vi "test2.vi"() -> ()   [LabVIEW 2025]
panel:
  out "x-y":u32
  out "Out":dbl
  in  "Boolean":bool
  in  "TC":dbl
  in  "IC Value":dbl
  in  "In":dbl
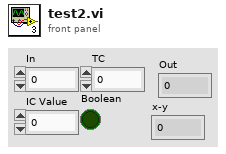
[diagram p1: front panel]
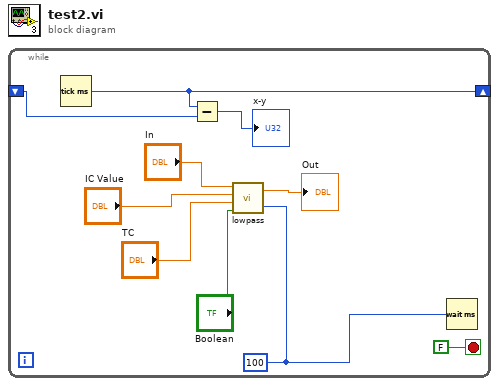
[diagram p0: block diagram]
diagram:
  n1 = while {
    shift-right: [w3] -> _
    shift-left: _ -> [w2]
    stop <- FALSE stop-if-true
    w4 = u32 100 ("milliseconds to wait")
    n2 = Tick Count (ms)() -> (millisecond timer value=w3:u32)
    n3 = Subtract(x=w3, y=w2) -> (x-y=→"x-y":u32)
    n4 = call "lowpass.vi"("MS"=w4, "Boolean"="Boolean", "TC"="TC", "IC Value"="IC Value", "In"="In") -> ("Out"=→"Out":dbl)
    n5 = Wait (ms)(milliseconds to wait=w4) -> ()  [unwired: 1 out]
  }
